vi "Value by Index.vi"(8 "error in (no error)":errorcluster, 10 "Index":i32, 11 "Group BOOL in":refnum<class "Group BOOL.lvclass">) -> (0 "error out":errorcluster, 1 "Timestamp":dbl, 2 "Scaled":bool, 3 "Group BOOL out":refnum<class "Group BOOL.lvclass">, 4 "Raw":bool)   [LabVIEW 2020, in "Vecto.lvlib" / "Group BOOL.lvclass"]
uses:
  Group BOOL.lvclass
  Group BOOL.lvclass/Group BOOL.ctl
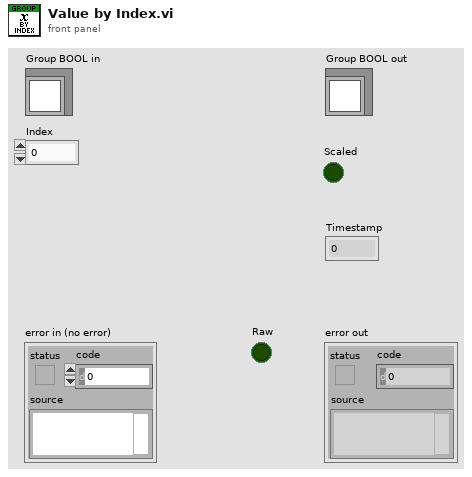
[diagram p1: front panel]
types:
  T1 = typedef "Vecto.lvlib/Group BOOL.lvclass/Ref.ctl" = cluster{"Scaled":bool[], "Timestamp":dbl[], "Raw":bool[]}
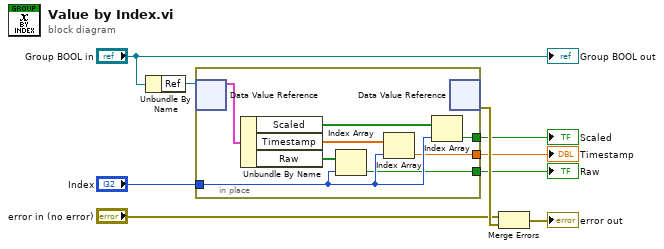
[diagram p0: block diagram]
diagram:
  n1 = Unbundle By Name("Group BOOL in") -> ("Ref"=w8:refnum<data-value>)
  n2 = in-place {
    in-place-border: "Index" -> [w13]
    in-place-border: [w12] -> w2
    in-place-border: [w11] -> w5
    in-place-border: [w10] -> w6
    n3 = in-place-dvr #1(w8) -> (w17:T1)  [unwired: 1 out]
    n4 = Unbundle By Name(w17) -> ("Scaled"=w14:bool[], "Timestamp"=w15:dbl[], "Raw"=w16:bool[])
    n5 = Index Array(array=w16, index=w13) -> (element=w12:bool)
    n6 = Index Array(array=w15, index=w13) -> (element=w11:dbl)
    n7 = Index Array(array=w14, index=w13) -> (element=w10:bool)
    n8 = in-place-dvr #1() -> (w9:errorcluster)  [unwired: 1 in, 1 out]
  }
  "Timestamp" <- w5
  "Scaled" <- w6
  "Raw" <- w2
  n9 = Merge Errors("error in (no error)", w9) -> (→"error out":errorcluster)
  "Group BOOL out" <- "Group BOOL in"
